vi "Voltage - On Demand Output.vi"() -> ()   [LabVIEW 2022 SP3]
doc: "This example demonstrates how to generate a user-defined voltage using the analog output of a DAQ device."
uses:
  <vilib>/Utility/error.llb/DialogType.ctl
  <vilib>/DAQmx/write.llb/DAQmx Write (Analog 1D DBL NChan 1Samp).vi
  <vilib>/DAQmx/create/channels.llb/DAQmx Create Channel (AO-Voltage-Basic).vi
  <vilib>/DAQmx/miscellaneous.llb/DAQmx Fill In Error Info.vi
panel:
  in  "Channel Array":dbl[](array[numeric])=[0.0]
  in  "Stop":bool
  in  "Max Voltage":dbl=10.0
  in  "Min Voltage":dbl=-10.0
  in  "Physical Channel(s)":tag="Dev1/ao0"
  # "Channel Settings"
  # "Output"
  # "The number of elements in the channel array\nmust equal the number of channels in the task."
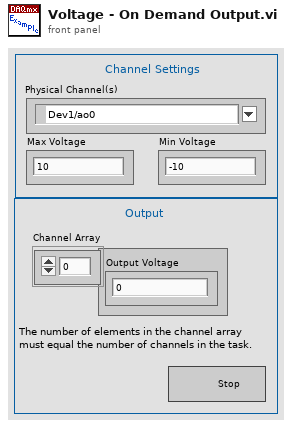
[diagram p1: front panel]
types:
  T1 = typedef "DialogType.ctl" = u16
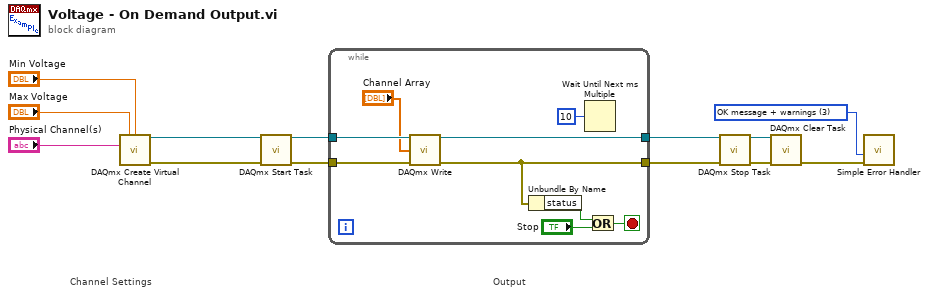
[diagram p0: block diagram]
diagram:
  w1 = T1 3 items=["no dialog", "OK message", "continue or stop message", "OK message + warnings", "continue/stop + warnings"] ("type of dialog (OK msg:1)")
  # "Output"
  # "Channel Settings"
  n1 = call-poly <vilib>:"DAQmx Create Virtual Channel.vi"("maximum value"="Max Voltage", "minimum value"="Min Voltage", "physical channels"="Physical Channel(s)") -> ("task out"=w9:refnum<k21>, "error out"=w8:errorcluster)  [unwired: 11 in]
  n2 = call <vilib>:"DAQmx Start Task.vi"("task/channels in"=w9, "error in"=w8) -> ("task out"=w7:refnum<k21>, "error out"=w6:errorcluster)  [unwired: 12 in]
  n3 = while {
    tunnel: w7 -> [w22]
    tunnel: w6 -> [w21]
    tunnel: [w16] -> w4
    tunnel: [w20] -> w5
    stop <- w15 stop-if-true
    n4 = call-poly <vilib>:"DAQmx Write.vi"("task/channels in"=w22, "data"="Channel Array", "error in"=w21) -> ("task out"=w20:refnum<k21>, "error out"=w16:errorcluster)  [unwired: 10 in, 1 out]
    n5 = Unbundle By Name(w16) -> ("status"=w18:bool)
    n6 = Wait Until Next ms Multiple(millisecond multiple=u32 10) -> ()  [unwired: 1 out]
    n7 = Or(x=w18, y="Stop") -> (x .or. y?=w15:bool)
  }
  n8 = call <vilib>:"DAQmx Stop Task.vi"("task/channels in"=w5, "error in"=w4) -> ("task out"=w3:refnum<k21>, "error out"=w2:errorcluster)  [unwired: 12 in]
  n9 = call <vilib>:"DAQmx Clear Task.vi"("task in"=w3, "error in"=w2) -> ("error out"=w13:errorcluster)  [unwired: 13 in]
  n10 = call <vilib>:"Simple Error Handler.vi"("type of dialog (OK msg:1)"=w1, "error in (no error)"=w13) -> ()  [unwired: 3 in, 5 out]
